vi "Get hard disk ID.vi"(8 "错误输入（无错误）":errorcluster, 10 "硬盘":enum16{"C", "D", "E", "F"}(ring)) -> (0 "错误输出":errorcluster, 2 "lpVolumeSerialNumber":u32)   [LabVIEW 2014]
uses:
  kernel32.dll
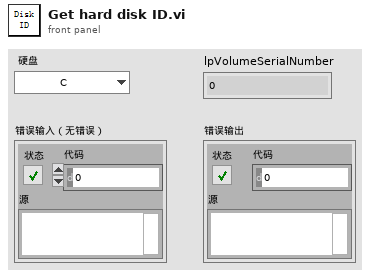
[diagram p1: front panel]
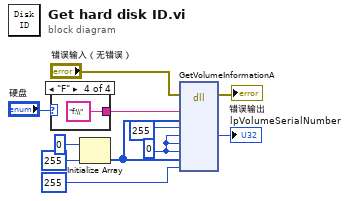
[diagram p0: block diagram]
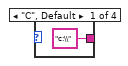
[diagram p2: hidden frame]
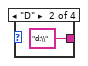
[diagram p3: hidden frame]
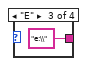
[diagram p4: hidden frame]
diagram:
  w8 = u32 0 ("lpRootPathName")
  n1 = case shown="\"F\"" "硬盘" {
    tunnel: ["c:\\" ("lpRootPathName") "d:\\" ("lpRootPathName") "e:\\" ("lpRootPathName") "f:\\" ("lpRootPathName")] -> w3
    frame "C", Default {
    }
    frame "D" {
    }
    frame "E" {
    }
    frame "F" {
    }
  }
  n2 = Initialize Array(u8 0, 255) -> (w6:u8[])
  n3 = dll-call lib="kernel32.dll" fn="GetVolumeInformationA"(error in="错误输入（无错误）", "lpRootPathName"=w3, "lpVolumeNameBuffer"=w6, "nVolumeNameSize"=u32 255, "lpVolumeSerialNumber"=w8, "lpMaximumComponentLength"=w8, "lpFileSystemFlags"=w8, "lpFileSystemNameBuffer"=w6, "nFileSystemNameSize"=u32 255) -> (error out=→"错误输出":errorcluster, "lpVolumeSerialNumber"=→"lpVolumeSerialNumber":u32)  [unwired: 10 in, 1 out]
